vi "Append Header, Footer and Watermark.vi"(0 "PDF Report IN":refnum<class "PDF Report Class.lvclass">, 11 "error in (no error)":errorcluster) -> (6 "Path":path, 15 "error out":errorcluster)   [LabVIEW 2019, in "Exaprom PDF.lvlib"]
doc: "Location: at the end of the report generation.\n\nThis can only be followed by \"Print PDF.vi\" and \"Dispose references.vi\".\n\nVersion 2.0\nDeveloped by Jean-Marc Simard\nCopyright © 2012, Exaprom Inc.\nAll rights reserved.\nLicense: BSD\n\nWith iTextSharp Library\n(http://itextsharp.sourceforge.net)"
uses:
  LV Class/PDF Report Class/PDF Report Class.lvclass
  Controls/Page Controls/Page dimensions.ctl
  Controls/Page Controls/Page Orientation.ctl
  Controls/Header, Footer and Watermark Controls/Header or Footer.ctl
  C:/work/niobrara_lv/labview pdf writer fixing/DLL/itextsharp.dll
  DLL/itextsharp.dll
  Exaprom PDF.lvlib
  LV Class/Fonts Class/Font Class.lvclass
  Controls/Page Controls/Page size.ctl
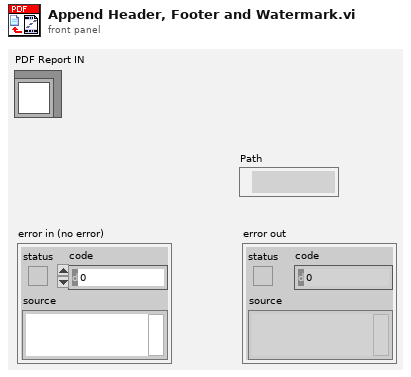
[diagram p1: front panel]
types:
  T1 = typedef "Exaprom PDF.lvlib/Page dimensions.ctl" = cluster{"Start at page":i32, "Page Size":T2, "Orientation":T3, "widht":sgl, "height":sgl, "Margin left":sgl, "Margin right":sgl, "Margin top":sgl, "Margin bottom":sgl, "X0":sgl, "X1":sgl, "Y0":sgl, "Y1":sgl}
  T2 = typedef "Exaprom PDF.lvlib/Page size.ctl" = i32
  T3 = typedef "Exaprom PDF.lvlib/Page Orientation.ctl" = enum16{"Portrait", "Landscape"}
  T4 = typedef "Exaprom PDF.lvlib/Header or Footer.ctl" = enum16{"Header", "Footer"}
  T5 = typedef "Exaprom PDF.lvlib/Watermark cluster2.ctl" = cluster{"Show? (F)":bool, "Type":enum16{"Image", "Text"}, "Opacity (%)":sgl, "Rotate(°)":sgl, "Position":cluster{"Position":T6, "X":sgl, "Y":sgl}, "Image path":path, "Scaled(%)":sgl, "Image refnum":refnum<k24>, "Text":string, "Font":cluster{"Name":string, "Size":T7, "Color":T8}, "Font refnum":refnum<k24>, "Alignment":T9, "Automatic":bool}
  T6 = typedef "Exaprom PDF.lvlib/Watermark Position.ctl" = enum16{"Absolute", "Center (page)", "Center (text section)"}
  T7 = typedef "Exaprom PDF.lvlib/Font size.ctl" = sgl
  T8 = typedef "Exaprom PDF.lvlib/Font color.ctl" = u32
  T9 = typedef "Exaprom PDF.lvlib/Header footer horiz alignment.ctl" = enum16{"Left", "Center", "Right"}
  T10 = typedef "Header Footer [ ] V2.ctl" = T11[]
  T11 = typedef "Header Footer cluster V2.ctl" = cluster{"Header or Footer":T4, "Start page":i32, "Start with #":i32, "Type":T12, "Alignment":T9, "Vertical Alignement":T13, "Line spacing":T14, "Image (%)":sgl, "Page #":T15, "Text":string, "Path":string, "Font":T16, "Font refnum":refnum<k24>, "Line":cluster{"Line":T19, "Thickness (points)":sgl, "Colour":T8}, "Vert margin":dbl, "Hyperlink":string}
  T12 = typedef "Exaprom PDF.lvlib/Header Footer Type.ctl" = enum16{"Select", "Text", "Text + hyperlink", "Page number", "Image", "Image + hyperlink"}
  T13 = typedef "Exaprom PDF.lvlib/Cell Vertical alignment.ctl" = enum16{"TOP", "MIDDLE", "BOTTOM"}
  T14 = typedef "Exaprom PDF.lvlib/Line spacing.ctl" = enum16{"Select", "1.0", "1.5", "2.0"}
  T15 = typedef "Exaprom PDF.lvlib/Page number.ctl" = cluster{"Text 1":string, "Text 2":string, "Text 3":string}
  T16 = typedef "Exaprom PDF.lvlib/Font complete cluster horizontal.ctl" = cluster{"Name":string, "Size":T7, "Color":T8, "Style":cluster{"Bold":bool, "Italic":bool, "Underline":bool, "Strikeout":bool}, "Type":T17}
  T17 = typedef "Exaprom PDF.lvlib/Type and encoding.ctl" = cluster{"Type&direction":T18, "Embedded":bool, "Encoding":string}
  T18 = typedef "Exaprom PDF.lvlib/Type and run direction.ctl" = enum16{"Select", "ASCII", "UTF-16", "UTF-16 (default)", "UTF-16 (LTR)", "UTF-16 (RTL)"}
  T19 = typedef "Exaprom PDF.lvlib/Header Footer Line.ctl" = enum16{"No line", "Horizontal line"}
  T20 = typedef "Exaprom PDF.lvlib/File Permission Parameters.ctl" = cluster{"User Password":string, "Owner Password":string, "Printing":enum16{"Allow Printing", "Allow Degraded Printing", "Don't Allow Printing"}, "Allow Modify Contents":bool, "Allow Copy":bool, "Allow Modify Annotations":bool, "Allow Fill In ":bool, "Allow Screen Readers":bool, "Allow Assembly":bool}
  T21 = typedef "Exaprom PDF.lvlib/Header Footer Complete Cluster.ctl" = cluster{"Table position":T22, "Header Footer Cluster with references [ ]":T23[]}
  T22 = typedef "Exaprom PDF.lvlib/Header or Footer Position.ctl" = cluster{"Vert margin":dbl, "FixedHeight":dbl, "Table X postion":dbl, "Table Y postion":dbl}
  T23 = typedef "Exaprom PDF.lvlib/Header Footer Cluster with references.ctl" = cluster{"Start page":i32, "Type":T12, "Start with #":i32, "Alignment":T9, "Vertical Alignement":T13, "Page #":T15, "Text":refnum<k24>, "Scaled Img":refnum<k24>, "PdfPCell":refnum<k24>, "PdfPTable":refnum<k24>, "Font Cluster":T16, "Font ":refnum<k24>, "Img (%)":sgl, "Line":cluster{"Line":T19, "Thickness (points)":sgl, "Colour":T8}, "Line spacing":T14}
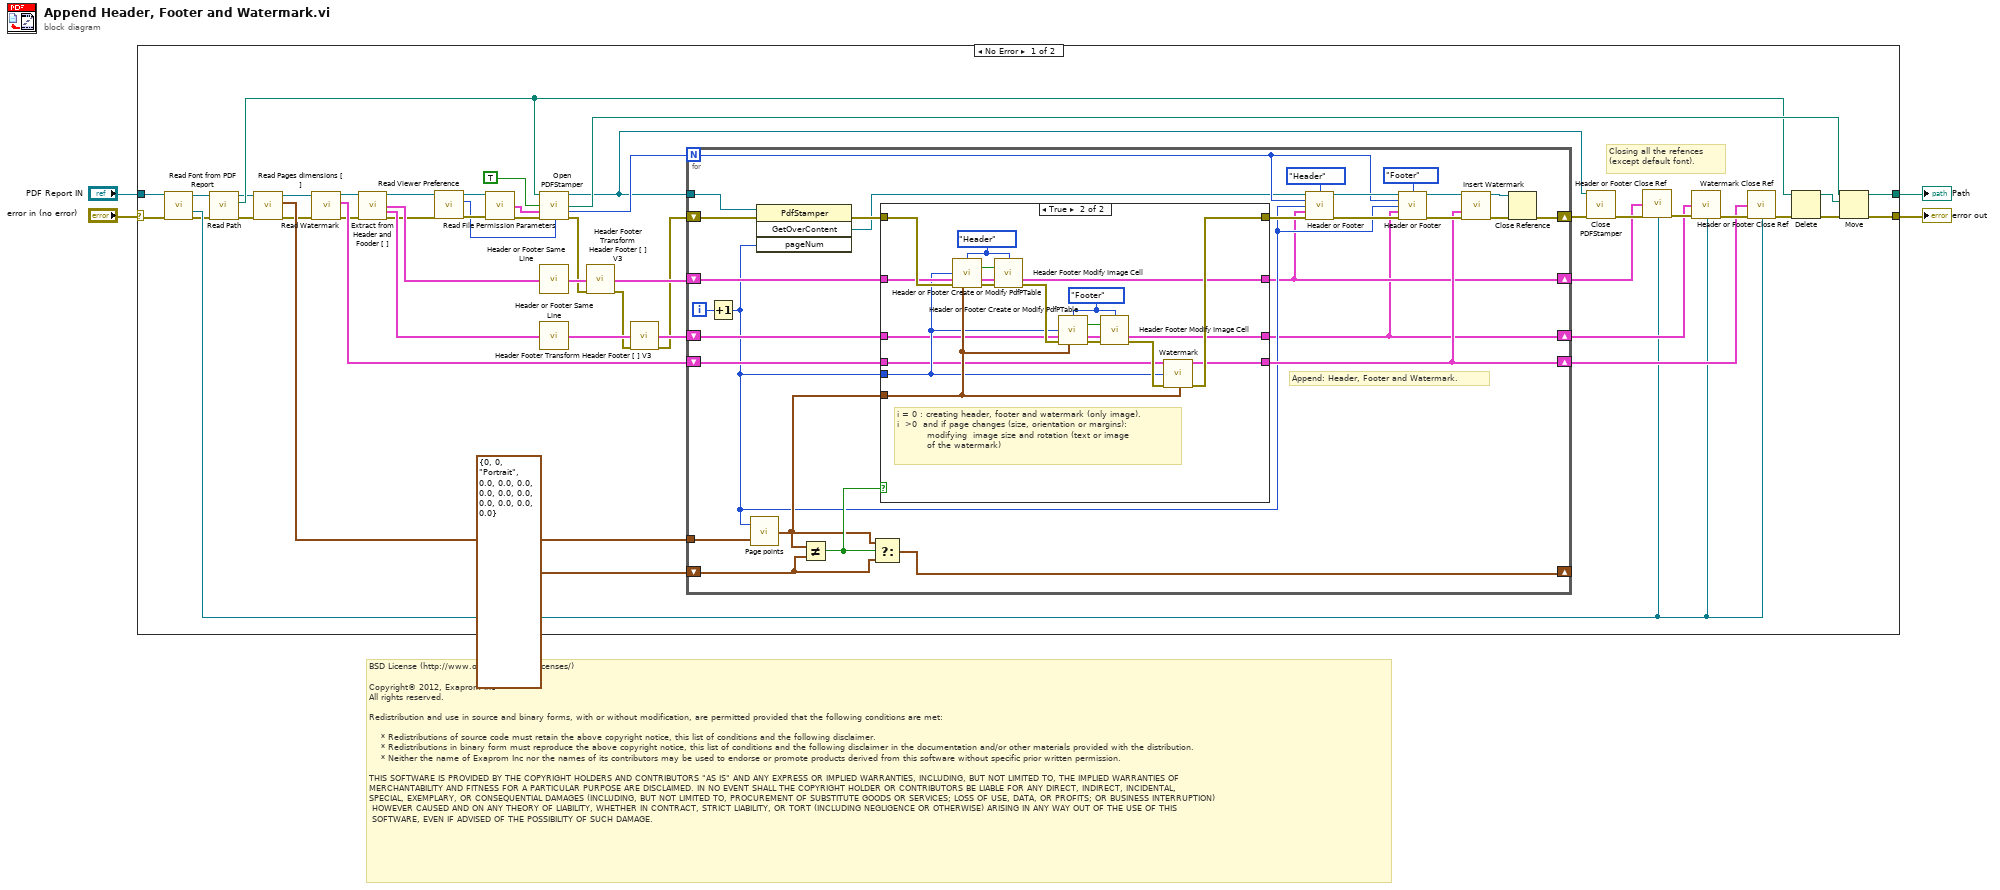
[diagram p0: block diagram]
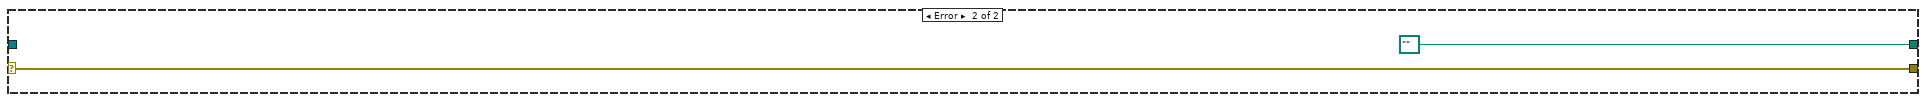
[diagram p3: hidden frame]
diagram:
  # "BSD License (http://www.opensource.org/licenses/)\n\nCopyright© 2012, Exaprom Inc\nAll rights reserved.\n\nRedistribution and use in source and binary forms, with or without modification, are permitted provided that the following conditions are met:\n\n    * Redistributions of source code must retain the above copyright notice, this list of conditions and the following disclaimer.\n    * Redistributions in binary form must reproduce the above copyright notice, this list of conditions and the following disclaimer in the documentation and/or other materials provided with the distribution.\n    * Neither the name of Exaprom Inc nor the names of its contributors may be used to endorse or promote products derived from this software without specific prior written permission.\n\nTHIS SOFTWARE IS PROVIDED BY THE COPYRIGHT HOLDERS AND CONTRIBUTORS \"AS IS\" AND ANY EXPRESS OR IMPLIED WARRANTIES, INCLUDING, BUT NOT LIMITED TO, THE IMPLIED WARRANTIES OF \nMERCHANTABILITY AND FITNESS FOR A PARTICULAR PURPOSE ARE DISCLAIMED. IN NO EVENT SHALL THE COPYRIGHT HOLDER OR CONTRIBUTORS BE LIABLE FOR ANY DIRECT, INDIRECT, INCIDENTAL,\nSPECIAL, EXEMPLARY, OR CONSEQUENTIAL DAMAGES (INCLUDING, BUT NOT LIMITED TO, PROCUREMENT OF SUBSTITUTE GOODS OR SERVICES; LOSS OF USE, DATA, OR PROFITS; OR BUSINESS INTERRUPTION)\n HOWEVER CAUSED AND ON ANY THEORY OF LIABILITY, WHETHER IN CONTRACT, STRICT LIABILITY, OR TORT (INCLUDING NEGLIGENCE OR OTHERWISE) ARISING IN ANY WAY OUT OF THE USE OF THIS\n SOFTWARE, EVEN IF ADVISED OF THE POSSIBILITY OF SUCH DAMAGE."
  n1 = case shown="No Error" "error in (no error)" {
    selector: "error in (no error)" -> [w14 w105]
    tunnel: [w28 w105] -> w4
    tunnel: "PDF Report IN" -> [w16 _]
    tunnel: [w51 path "" ("new path")] -> w1
    frame No Error {
      # "Closing all the refences \n(except default font)."
      n2 = call "Read Font from PDF Report.vi"("PDF Report"=w16, "error in (no error)"=w14) -> ("PDF Report duplicate"=w15:refnum<class "PDF Report Class.lvclass">, "Font Ref"=w24:refnum<k24>, "error out"=w17:errorcluster)  [unwired: 7 in, 4 out]
      n3 = call-dynamic "Read Path.vi"("error in (no error)"=w17, "PDF Report Class in"=w15) -> ("error out"=w18:errorcluster, "Path"=w27:path, "PDF Report Class out"=w19:refnum<class "PDF Report Class.lvclass">)  [unwired: 7 in]
      n4 = call-dynamic "Read Pages dimensions [ ].vi"("error in (no error)"=w18, "PDF Report Class in"=w19) -> ("error out"=w21:errorcluster, "Pages dimensions [ ]"=w26:T1[], "PDF Report Class out"=w20:refnum<class "PDF Report Class.lvclass">)  [unwired: 6 in, 1 out]
      n5 = call-dynamic "Read Watermark .vi"("error in (no error)"=w21, "PDF Report Class in"=w20) -> ("error out"=w23:errorcluster, "Watermark Cluster"=w25:T5, "PDF Report Class out"=w22:refnum<class "PDF Report Class.lvclass">)  [unwired: 7 in]
      n6 = call "Extract from Header and Fooder [ ].vi"("PDF Report IN"=w22, "error in (no error)"=w23) -> ("PDF Report OUT"=w10:refnum<class "PDF Report Class.lvclass">, "Header [ ]"=w13:T10, "Footer [ ]"=w12:T10, "error out"=w7:errorcluster)  [unwired: 9 in, 1 out]
      n7 = call-dynamic "Read Viewer Preference.vi"("error in (no error)"=w7, "PDF Report Class in"=w10) -> ("error out"=w6:errorcluster, "Viewer Preference"=w5:u16, "PDF Report Class out"=w8:refnum<class "PDF Report Class.lvclass">)  [unwired: 7 in]
      n8 = call-dynamic "Read File Permission Parameters.vi"("PDF Report Class in"=w8, "error in (no error)"=w6) -> ("File Permission Parameters"=w9:T20, "error out"=w11:errorcluster)  [unwired: 11 in, 1 out]
      n9 = call "Open PDFStamper.vi"("PDF Path (original)"=w27, "RotateContents (F)"=TRUE, "Permissions"=w9, "error in (no error)"=w11, "Viewer Preference"=w5) -> ("PDFStamper"=w41:refnum<k24>, "Temporary File Name"=w47:path, "NumberOfPages"=w49:i32, "error out"=w35:errorcluster)  [unwired: 2 in, 5 out]
      n10 = call "Header or Footer Same Line.vi"("Header Footer [ ] IN"=w13) -> ("Header Footer [ ] OUT"=w40:T10)
      n11 = call "Header or Footer Same Line.vi"("Header Footer [ ] IN"=w12) -> ("Header Footer [ ] OUT"=w38:T10)
      n12 = call "Header Footer Transform Header Footer [ ] V3.vi"("Header or Footer [ ]"=w40, "error in (no error)"=w35) -> ("Header or Footer Complete Cluster"=w39:T21, "error out"=w36:errorcluster)  [unwired: 12 out]
      n13 = call "Header Footer Transform Header Footer [ ] V3.vi"("Header or Footer [ ]"=w38, "error in (no error)"=w36) -> ("Header or Footer Complete Cluster"=w37:T21, "error out"=w34:errorcluster)  [unwired: 12 out]
      n14 = for {
        N: w49 -> [w67]
        tunnel: w41 -> [w73]
        tunnel: w26 -> [w68]
        shift-right: [w66] -> _
        shift-left: T1 {"Start at page"=0, "Page Size"=0, "Orientation"=enum."Portrait", "widht"=0.0, "height"=0.0, "Margin left"=0.0, "Margin right"=0.0, "Margin top"=0.0, "Margin bottom"=0.0, "X0"=0.0, "X1"=0.0, "Y0"=0.0, "Y1"=0.0} ("Page (points)") -> [w65]
        shift-right: [w60] -> w29
        shift-left: w25 -> [w59]
        shift-right: [w58] -> w48
        shift-left: w34 -> [w74]
        shift-right: [w54] -> w33
        shift-left: w39 -> [w63]
        shift-right: [w53] -> w32
        shift-left: w37 -> [w61]
        i -> [w75]
        # "Append: Header, Footer and Watermark."
        n15 = Increment(x=w75) -> (x+1=w55:i32)
        n16 = call "Page points.vi"("Pages dimensions [ ]"=w68, "pageNum"=w55) -> ("Page (points)"=w62:T1)
        n17 = invoke class="PdfStamper" method="GetOverContent"(reference=w73, error in=w74, "pageNum"=w55) -> (error out=w78:errorcluster, "GetOverContent"=w52:refnum<k24>)  [unwired: 1 in, 2 out]
        n18 = Not Equal?(x=w62, y=w65) -> (x != y?=w64:bool)
        n19 = Select(t=w62, s=w64, f=w65) -> (s? t:f=w66:T1)
        n20 = case shown="True" w64 {
          tunnel: w63 -> [w82 w99]
          tunnel: w62 -> [_ w95]
          tunnel: w61 -> [w81 w86]
          tunnel: w78 -> [w80 w103]
          tunnel: [w80 w101] -> w79
          tunnel: w59 -> [w83 w91]
          tunnel: [w83 w96] -> w60
          tunnel: w55 -> [_ w94]
          tunnel: [w82 w88] -> w54
          tunnel: [w81 w87] -> w53
          frame False {
          }
          frame True {
            w92 = Header_or_Footer."Footer" ("Header or Footer")
            w93 = Header_or_Footer."Header" ("Header or Footer")
            # "i = 0 : creating header, footer and watermark (only image).\ni  >0  and if page changes (size, orientation or margins):\n          modifying  image size and rotation (text or image \n          of the watermark)"
            n21 = call "Header or Footer Create or Modify PdfPTable.vi"("Header or Footer"=w93, "pageNum"=w94, "Header Footer IN [ ]"=w99, "error in (no error)"=w103, "Page points"=w95) -> ("Modify Image Cell"=w85:bool, "Header Footer OUT [ ]"=w89:T21, "error out"=w98:errorcluster)  [unwired: 3 in, 5 out]
            n22 = call "Header Footer Modify Image Cell.vi"("Header or Footer"=w93, "Modify Image Cell"=w85, "Header or Footer Complete Cluster IN"=w89, "error in (no error)"=w98) -> ("Header or Footer Complete Cluster OUT"=w88:T21, "error out"=w100:errorcluster)  [unwired: 1 in, 9 out]
            n23 = call "Header or Footer Create or Modify PdfPTable.vi"("Header or Footer"=w92, "pageNum"=w94, "Header Footer IN [ ]"=w86, "error in (no error)"=w100, "Page points"=w95) -> ("Modify Image Cell"=w84:bool, "Header Footer OUT [ ]"=w90:T21, "error out"=w97:errorcluster)  [unwired: 3 in, 5 out]
            n24 = call "Header Footer Modify Image Cell.vi"("Header or Footer"=w92, "Modify Image Cell"=w84, "Header or Footer Complete Cluster IN"=w90, "error in (no error)"=w97) -> ("Header or Footer Complete Cluster OUT"=w87:T21, "error out"=w102:errorcluster)  [unwired: 1 in, 9 out]
            n25 = call "Watermark.vi"("Watermark IN"=w91, "pageNum"=w94, "error in (no error)"=w102, "Page dimensions"=w95) -> ("Watermark OUT"=w96:T5, "error out"=w101:errorcluster)  [unwired: 2 in, 8 out]
          }
        }
        n26 = call "Header or Footer.vi"("OverContent"=w52, "Header or Footer"=Header_or_Footer."Header", "NumberOfPages"=w67, "pageNum"=w55, "Header or Footer Complete Cluster"=w54, "error in (no error)"=w79) -> ("OverContent duplicate"=w76:refnum<k24>, "error out"=w77:errorcluster)  [unwired: 2 in, 6 out]
        n27 = call "Header or Footer.vi"("OverContent"=w76, "Header or Footer"=Header_or_Footer."Footer", "NumberOfPages"=w67, "pageNum"=w55, "Header or Footer Complete Cluster"=w53, "error in (no error)"=w77) -> ("OverContent duplicate"=w71:refnum<k24>, "error out"=w72:errorcluster)  [unwired: 1 in, 7 out]
        n28 = call "Insert Watermark.vi"("OverContent"=w71, "Watermark Cluster"=w60, "error in (no error)"=w72) -> ("OverContent duplicate"=w69:refnum<k24>, "error out"=w70:errorcluster)  [unwired: 3 in, 8 out]
        n29 = Close Reference(reference=w69, error in (no error)=w70) -> (error out=w58:errorcluster)
      }
      n30 = call "Close PDFStamper.vi"("PDFStamper"=w41, "error in (no error)"=w48) -> ("error out"=w43:errorcluster)  [unwired: 13 out]
      n31 = call "Header or Footer Close Ref.vi"("Header or Footer Complete Cluster"=w33, "error in (no error)"=w43, "Default Font"=w24) -> ("error out"=w42:errorcluster)  [unwired: 1 in, 11 out]
      n32 = call "Header or Footer Close Ref.vi"("Header or Footer Complete Cluster"=w32, "error in (no error)"=w42, "Default Font"=w24) -> ("error out"=w31:errorcluster)  [unwired: 12 out]
      n33 = call "Watermark Close Ref.vi"("Watermark IN"=w29, "error in (no error)"=w31, "Default Font"=w24) -> ("error out"=w30:errorcluster)  [unwired: 12 out]
      n34 = Delete(path (use dialog)=w27, error in=w30) -> (deleted path=w45:path, error out=w44:errorcluster)  [unwired: 4 out]
      n35 = Move(source path=w47, error in=w44, 10:w45) -> (error out=w28:errorcluster, 3:w51:path)  [unwired: 3 out]
    }
    frame Error {
    }
  }
  "error out" <- w4
  "Path" <- w1
